vi "Configuration_Ref_API.vi"(0 "DVR In":refnum<data-value>, 11 "Error In":errorcluster) -> (4 "DVR Out":refnum<data-value>, 6 "VI Ref":refnum<vi>, 15 "Error Out":errorcluster)   [LabVIEW 2020, in "Test.lvclass"]
doc: "Configuration Reference API"
uses:
  Test.lvclass
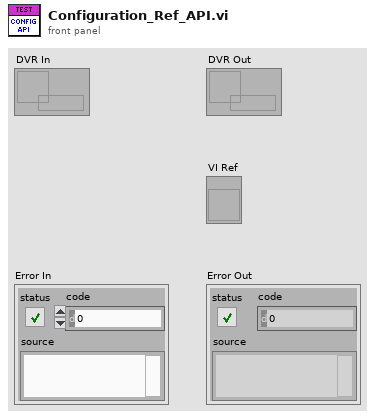
[diagram p1: front panel]
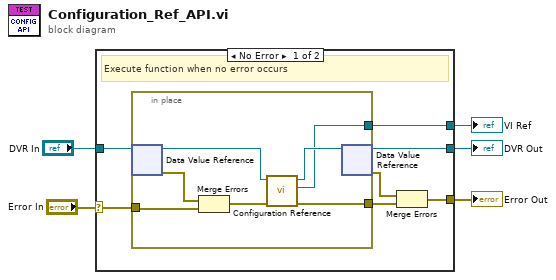
[diagram p0: block diagram]
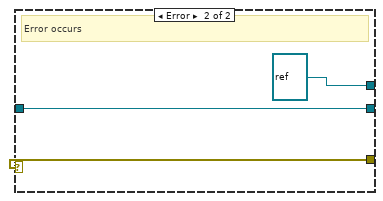
[diagram p2: hidden frame]
diagram:
  n1 = case shown="No Error" "Error In" {
    selector: "Error In" -> [w11 w22]
    tunnel: "DVR In" -> [w12 w21]
    tunnel: [w10 refnum<vi> refnum ("VI Ref")] -> w3
    tunnel: [w9 w21] -> w2
    tunnel: [w6 w22] -> w1
    frame No Error {
      # "Execute function when no error occurs"
      n2 = in-place {
        in-place-border: w11 -> [w19]
        in-place-border: [w14] -> w10
        in-place-border: [w13] -> w7
        n3 = in-place-dvr #1(w12) -> (w16:refnum<class "Test.lvclass">, w18:errorcluster)
        n4 = Merge Errors(w18, w19) -> (w17:errorcluster)
        n5 = call-dynamic "Configuration Reference.vi"("Error in"=w17, "Test in"=w16) -> ("Error out"=w13:errorcluster, "VI Ref"=w14:refnum<vi>, "Test out"=w15:refnum<class "Test.lvclass">)  [unwired: 7 in]
        n6 = in-place-dvr #1(w15) -> (w9:refnum<data-value>, w8:errorcluster)
      }
      n7 = Merge Errors(w8, w7) -> (w6:errorcluster)
    }
    frame Error {
      # "Error occurs"
    }
  }
  "VI Ref" <- w3
  "DVR Out" <- w2
  "Error Out" <- w1
